vi "ConvertZAxisToX.vi"(7 "Axis in":enum16{"Z", "Y", "X"}(ring)) -> (3 "Axis out":enum16{"Z", "Y", "X"}(ring))   [LabVIEW 2023]
doc: "Convert the Z axis enum value to X"
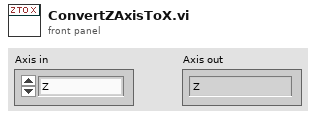
[diagram p1: front panel]
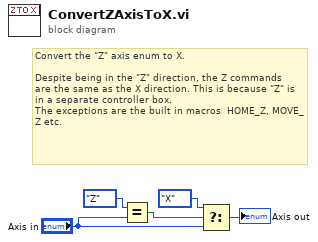
[diagram p0: block diagram]
diagram:
  # "Convert the \"Z\" axis enum to X. \n\nDespite being in the \"Z\" direction, the Z commands\nare the same as the X direction. This is because \"Z\" is in a separate controller box.\nThe exceptions are the built in macros  HOME_Z, MOVE_Z etc."
  n1 = Equal?(x=enum16{"Z", "Y", "X"}."Z" ("y"), y="Axis in") -> (x = y?=w4:bool)
  n2 = Select(t=enum16{"Z", "Y", "X"}."X" ("y"), s=w4, f="Axis in") -> (s? t:f=→"Axis out":enum16{"Z", "Y", "X"})
